vi "step4 TestAndSolveUpperCross.vi"(11 "cube in":T1) -> (3 "cube out":T1)   [LabVIEW 2011]
uses:
  Typedef/cube.ctl
  Typedef/face.ctl
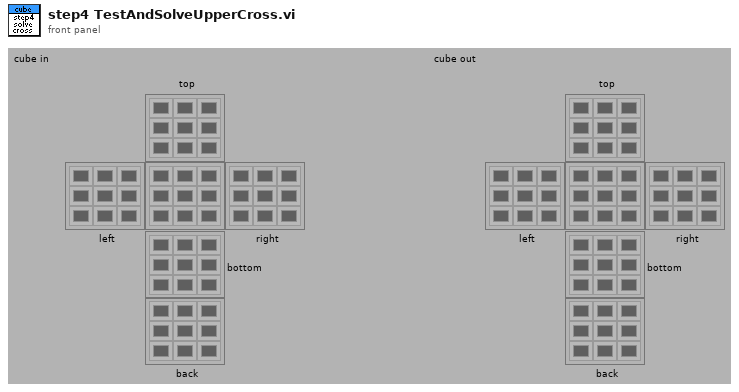
[diagram p1: front panel]
types:
  T1 = typedef "cube.ctl" = cluster{"top":T2, "left":T2, "right":T2, "bottom":T2, "back":T2, "front":T2}
  T2 = typedef "face.ctl" = u32[][]
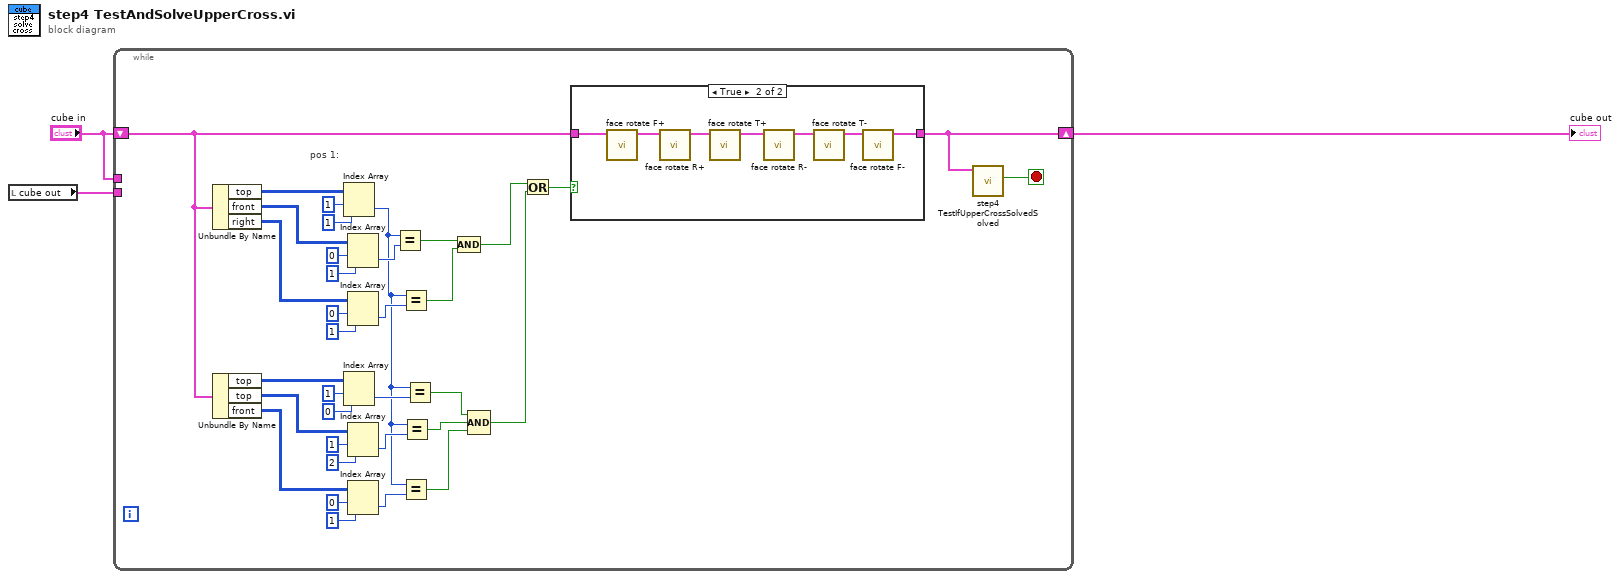
[diagram p0: block diagram]
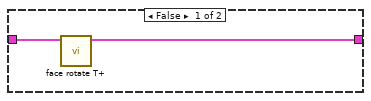
[diagram p2: hidden frame]
diagram:
  n1 = local read "cube out"() -> (w2:T1)
  n2 = while {
    shift-right: [w4] -> w1
    shift-left: "cube in" -> [w6]
    tunnel: "cube in" -> [_]
    tunnel: w2 -> [_]
    stop <- w5 stop-if-true
    # "pos 1:"
    n3 = Unbundle By Name(w6) -> ("top"=w34:T2, "front"=w36:T2, "right"=w29:T2)
    n4 = Unbundle By Name(w6) -> ("top"=w21:T2, "top"=w19:T2, "front"=w25:T2)
    n5 = Index Array(array=w34, index (row)=1, index (col)=1 ("disabled index (col)")) -> (element=w11:u32)
    n6 = Index Array(array=w21, index (row)=1, index (col)=0 ("disabled index (col)")) -> (element=w15:u32)
    n7 = Index Array(array=w36, index (row)=0, index (col)=1 ("disabled index (col)")) -> (element=w32:u32)
    n8 = Index Array(array=w29, index (row)=0, index (col)=1 ("disabled index (col)")) -> (element=w28:u32)
    n9 = Index Array(array=w19, index (row)=1, index (col)=2 ("disabled index (col)")) -> (element=w16:u32)
    n10 = Index Array(array=w25, index (row)=0, index (col)=1 ("disabled index (col)")) -> (element=w10:u32)
    n11 = Equal?(x=w11, y=w32) -> (x = y?=w27:bool)
    n12 = Equal?(x=w11, y=w28) -> (x = y?=w26:bool)
    n13 = Equal?(x=w11, y=w10) -> (x = y?=w12:bool)
    n14 = Equal?(x=w11, y=w16) -> (x = y?=w13:bool)
    n15 = Equal?(x=w11, y=w15) -> (x = y?=w14:bool)
    n16 = Compound Arithmetic op=AND(w27, w26) -> (w9:bool)
    n17 = Compound Arithmetic op=AND(w14, w13, w12) -> (w8:bool)
    n18 = Or(x=w9, y=w8) -> (x .or. y?=w7:bool)
    n19 = case shown="True" w7 {
      tunnel: w6 -> [w40 w47]
      tunnel: [w39 w41] -> w4
      frame False {
        n20 = call "face rotate T+.vi"("cube in"=w40) -> ("cube out"=w39:T1)  [unwired: 9 in, 1 out]
      }
      frame True {
        n21 = call "face rotate F+.vi"("cube in"=w47) -> ("cube out"=w46:T1)  [unwired: 9 in, 1 out]
        n22 = call "face rotate R+.vi"("cube in"=w46) -> ("cube out"=w45:T1)  [unwired: 9 in, 1 out]
        n23 = call "face rotate T+.vi"("cube in"=w45) -> ("cube out"=w44:T1)  [unwired: 9 in, 1 out]
        n24 = call "face rotate R-.vi"("cube in"=w44) -> ("cube out"=w43:T1)  [unwired: 9 in, 1 out]
        n25 = call "face rotate T-.vi"("cube in"=w43) -> ("cube out"=w42:T1)  [unwired: 9 in, 1 out]
        n26 = call "face rotate F-.vi"("cube in"=w42) -> ("cube out"=w41:T1)  [unwired: 9 in, 1 out]
      }
    }
    n27 = call "step4 TestIfUpperCrossSolvedSolved.vi"("cube in"=w4) -> ("upper cross solved?"=w5:bool)  [unwired: 9 in, 1 out]
  }
  "cube out" <- w1
